vi "SoundRecorderMATLAB.vi"() -> ()   [LabVIEW 2012]
uses:
  <vilib>/Waveform/WDTOps.llb/WDT Get Waveform Time Array DBL.vi
  <vilib>/Utility/file.llb/Write To Spreadsheet File (DBL).vi
panel:
  in  "Sampling Rate":dbl
  in  "Sample Time":dbl
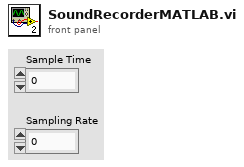
[diagram p1: front panel]
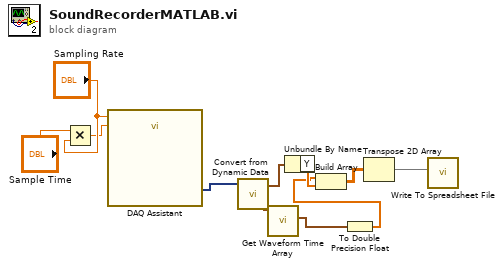
[diagram p0: block diagram]
diagram:
  n1 = Multiply(x="Sample Time", y="Sampling Rate") -> (x*y=w8:dbl)
  n2 = call "DAQ Assistant"("rate"="Sampling Rate", "number of samples"=w8) -> ("data"=w7:dynamicdata)  [unwired: 15 in, 2 out]
  n3 = call "Convert from Dynamic Data"("Dynamic Data Type"=w7) -> ("Waveform"=w6:waveform(dbl))  [unwired: 3 in]
  n4 = call-poly <vilib>:"Get Waveform Time Array.vi"("waveform in"=w6) -> ("X array"=w5:timestamp[])  [unwired: 9 in, 1 out]
  n5 = Unbundle By Name(w6) -> ("Y"=w2:dbl[])
  n6 = To Double Precision Float(number=w5) -> (double precision float=w1:dbl[])
  n7 = Build Array(w1, w2) -> (w4:dbl[][])
  n8 = Transpose 2D Array(2D array=w4) -> (transposed array=w3:dbl[][])
  n9 = call-poly <vilib>:"Write To Spreadsheet File.vi"("2D data"=w3) -> ()  [unwired: 7 in, 1 out]
